vi "writeToXML.vi"(8 "error in (no error)":errorcluster, 10 "ClassLabel":string, 11 "GuideTargetOffset in":refnum<class "GuideTargetOffset.lvclass">) -> (0 "error out":errorcluster, 2 "XML out":string, 3 "GuideTargetOffset out":refnum<class "GuideTargetOffset.lvclass">)   [LabVIEW 2014, in "TCSDataDefinitions.lvlib" / "TCSCommand.lvlib" / "OffsetCommands.lvlib" / "GuideTargetOffset.lvclass"]
uses:
  GuideTargetOffset.lvclass
  Offset/Offset.lvclass
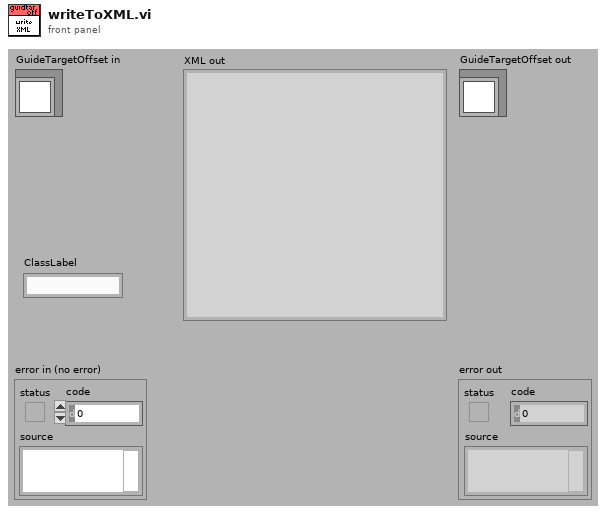
[diagram p1: front panel]
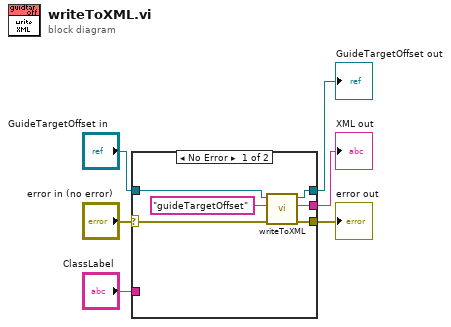
[diagram p0: block diagram]
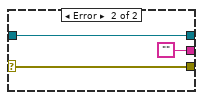
[diagram p2: hidden frame]
diagram:
  n1 = case shown="No Error" "error in (no error)" {
    selector: "error in (no error)" -> [w12 w15]
    tunnel: [w11 w15] -> w5
    tunnel: [w8 w14] -> w3
    tunnel: "GuideTargetOffset in" -> [w9 w14]
    tunnel: [w10 ""] -> w2
    tunnel: "ClassLabel" -> [_ _]
    frame No Error {
      n2 = call-parent "writeToXML.vi"("error in (no error)"=w12, "ClassLabel"="guideTargetOffset", "Offset in"=w9) -> ("error out"=w11:errorcluster, "XML out"=w10:string, "Offset out"=w8:refnum<class "GuideTargetOffset.lvclass">)  [unwired: 6 in]
    }
    frame Error {
    }
  }
  "error out" <- w5
  "GuideTargetOffset out" <- w3
  "XML out" <- w2
